vi "meas_cycle_TD_FFT.vi"(2 "chirp end":dbl, 3 "time domain array":dbl[](array[numeric]), 4 "dt":dbl, 5 "current frequency":dbl) -> (0 "output time domain signal":waveform(dbl), 1 "output spectrum":T1)   [LabVIEW 2011]
doc: "converts the time domain data to freq. domain data and corrects the frequency offset. \n\nFurthermore, the DC component is deleted from the freq. domain signal."
uses:
  <vilib>/express/express analysis/Spectral/Block/exnSpectralBlock spectral measurements power poly.vi
  <vilib>/express/express analysis/Spectral/Block/exnSpectralBlock spectral measurements power WFM.vi
  <vilib>/express/express analysis/Spectral/XNode/ExpressSpectralMeasurementsBlockNode.xnode
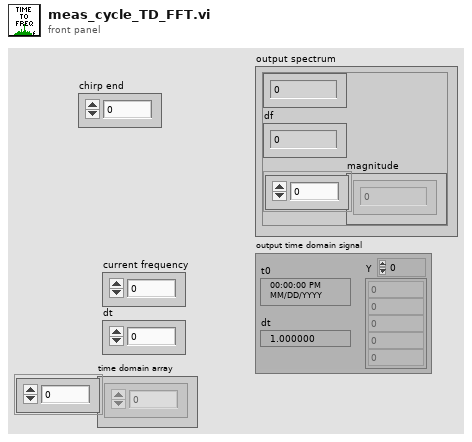
[diagram p1: front panel]
types:
  T1 = cluster{"Numeric Control":dbl, "df":dbl, "magnitude":dbl[]}
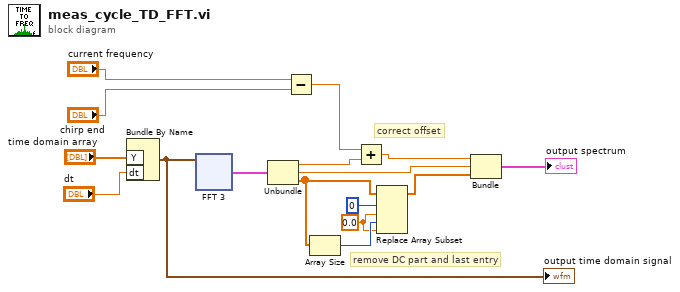
[diagram p0: block diagram]
diagram:
  w9 = 0.0 ("new element/subarray")
  # "remove DC part and last entry"
  # "correct offset"
  n1 = Bundle By Name("Y"="time domain array", "dt"="dt") -> (w14:waveform(dbl))  [unwired: 1 in]
  "output time domain signal" <- w14
  n2 = xnode ("FFT 3")("Signals"=w14) -> ("Power Spectrum"=w15:cluster{"f0":dbl, "df":dbl, "magnitude":dbl[]})  [unwired: 1 in, 1 out]
  n3 = Unbundle(w15) -> ("f0"=w3:dbl, "df"=w8:dbl, "magnitude"=w11:dbl[])
  n4 = Subtract(x="current frequency", y="chirp end") -> (x-y=w2:dbl)
  n5 = Array Size(array=w11) -> (size(s)=w10:i32)
  n6 = Add(x=w2, y=w3) -> (x+y=w1:dbl)
  n7 = Replace Array Subset(array=w11, new element #1=w9, index #1=0 ("index"), new element #2=w9, index #2=w10) -> (w7:dbl[])
  n8 = Bundle(w1, "df"=w8, "magnitude"=w7) -> (→"output spectrum":cluster{dbl, "df":dbl, "magnitude":dbl[]})  [unwired: 1 in]
